vi "printLastLines.vi"(10 "Number of lines to show":i32=4, 11 "Inserted string":string) -> (3 "Last lines":string[](array[string]))   [LabVIEW 2017]
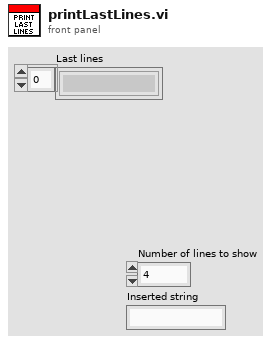
[diagram p1: front panel]
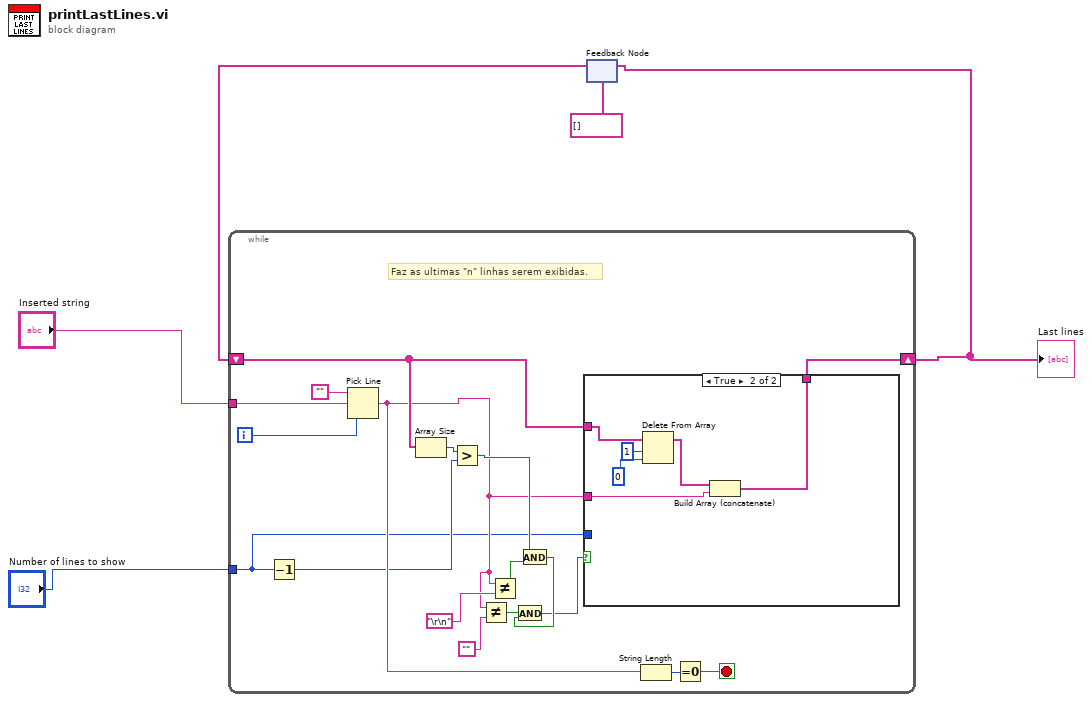
[diagram p0: block diagram]
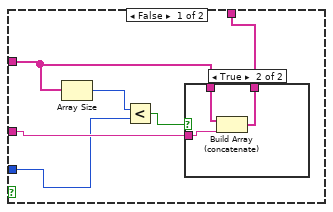
[diagram p2: hidden frame]
diagram:
  n1 = feedback #1(string[] []) -> (w5:string[])
  n2 = while {
    shift-right: [w13] -> w4
    shift-left: w5 -> [w17]
    tunnel: "Inserted string" -> [w19]
    tunnel: "Number of lines to show" -> [w6]
    i -> [w23]
    stop <- w20 stop-if-true
    # "Faz as ultimas \"n\" linhas serem exibidas."
    n3 = Decrement(x=w6) -> (x-1=w7:i32)
    n4 = Pick Line(string ("")="", multi-line string=w19, line index=w23) -> (output string=w10:string)
    n5 = Array Size(array=w17) -> (size(s)=w18:i32)
    n6 = Greater?(x=w18, y=w7) -> (0:w16:bool)
    n7 = Not Equal?(x=w10, y="") -> (x != y?=w12:bool)
    n8 = Not Equal?(x=w10, y="\r\n") -> (x != y?=w15:bool)
    n9 = And(x=w16, y=w15) -> (x .and. y?=w9:bool)
    n10 = And(x=w12, y=w9) -> (x .and. y?=w8:bool)
    n11 = case shown="True" w8 {
      tunnel: w17 -> [w27 w37]
      tunnel: [w25 w38] -> w13
      tunnel: w10 -> [w26 w39]
      tunnel: w6 -> [w24 _]
      frame False {
        n12 = Array Size(array=w27) -> (size(s)=w29:i32)
        n13 = Less?(x=w29, y=w24) -> (x < y?=w28:bool)
        n14 = case shown="True" w28 {
          tunnel: w27 -> [w30 w33]
          tunnel: w26 -> [_ w32]
          tunnel: [w30 w31] -> w25
          frame False {
          }
          frame True {
            n15 = Build Array (concatenate)(w33, w32) -> (w31:string[])
          }
        }
      }
      frame True {
        n16 = Delete From Array(array=w37, length=1, index=0) -> (array with subset deleted=w34:string[])  [unwired: 1 out]
        n17 = Build Array (concatenate)(w34, w39) -> (w38:string[])
      }
    }
    n18 = String Length(string=w10) -> (length=w21:i32)
    n19 = Equal To 0?(x=w21) -> (x = 0?=w20:bool)
  }
  "Last lines" <- w4
  n20 = feedback-in #1(w4) -> ()
